vi "Reaction.vi"(8 "Size (m)":cluster{"Width":sgl, "Height":sgl}={"Width"=nan, "Height"=nan} caption="Size (m) (NaN=no change)" {"Height" format="%.2p"; "Width" format="%.2p"}, 9 "Center coordinates (m)":cluster{"Xc":sgl, "Yc":sgl}={"Xc"=nan, "Yc"=nan} caption="Center coordinates (m) (NaN=no change)" {"Yc" format="%.2p"; "Xc" format="%.2p"}, 10 "XYData":sgl[][](array[numeric]) format="%#_5p", 11 "Application ref in":refnum<vi>) -> (0 "rollout":dbl[](array[numeric]), 1 "Boolean":bool, 2 "Data":sgl[][](array[numeric]) format="%#_5p", 3 "Application ref out":refnum<vi>)   [LabVIEW 2020]
uses:
  <userlib>/Nanonis Prog Interface V5/Nanonis Prog Interface.lvlib
panel:
  in  "array 2":dbl[](array[numeric])=[1.0, 2.0]
  in  "Python version":string="3.6"
  in  "module path":path=path "D:/Git repo/pythonProject/STM_Python_Modules/RxnClass.py"
  in  "Python version 4":string="3.6"
  in  "module path 4":path=path "D:/Git repo/pythonProject/STM_Python_Modules/KpDet.py"
  in  "array":dbl[](array[numeric])=[1.0, 2.0]
  out "Error out":errorcluster
  in  "error in (no error)":errorcluster
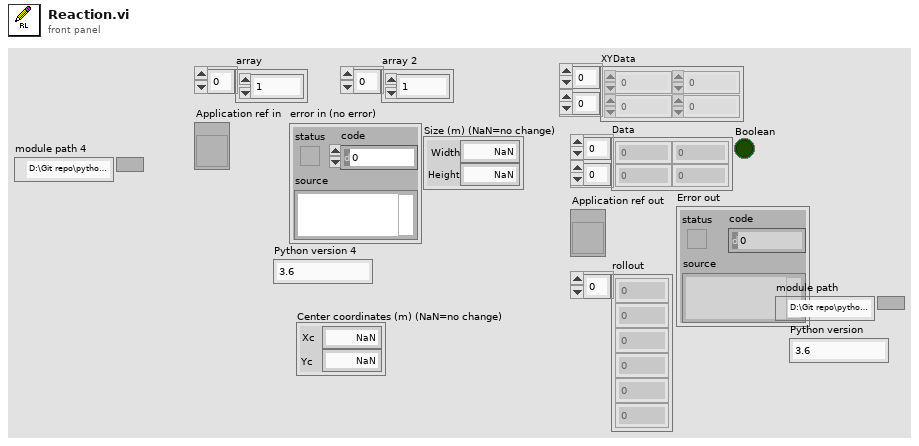
[diagram p1: front panel]
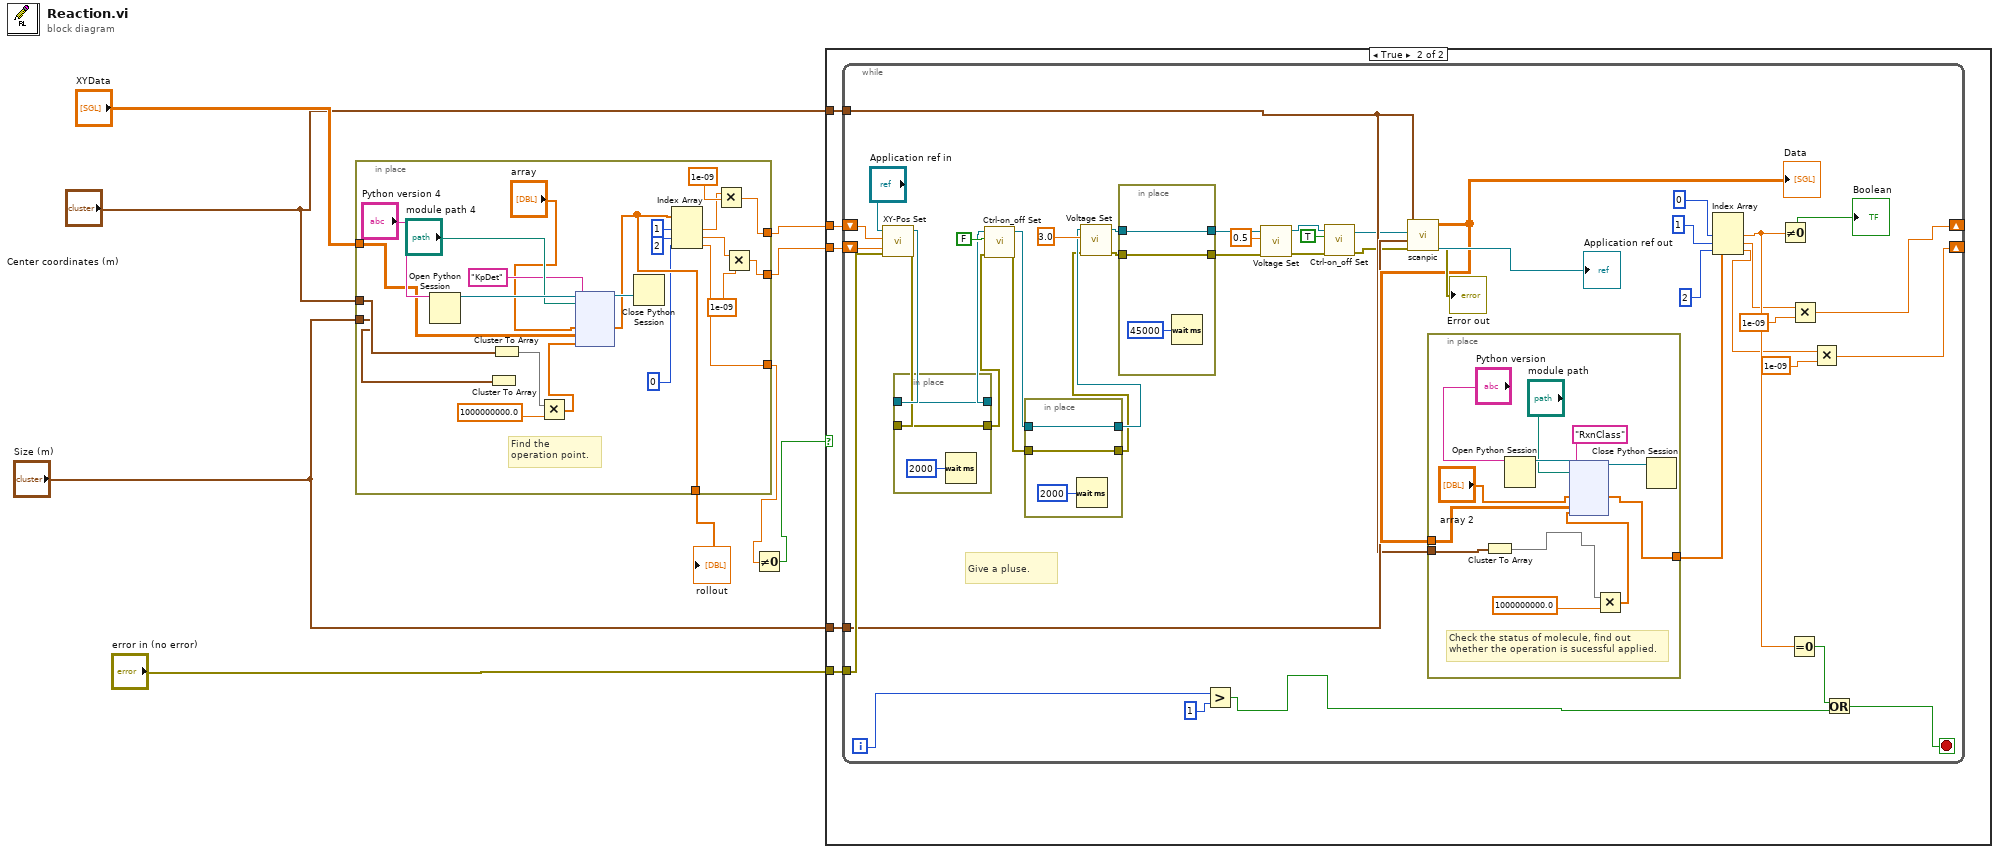
[diagram p0: block diagram]
diagram:
  n1 = in-place {
    in-place-border: "XYData" -> [w24]
    in-place-border: "Size (m)" -> [w21]
    in-place-border: [w13] -> w4
    in-place-border: [w10] -> w3
    in-place-border: [w23] -> w6
    in-place-border: "Center coordinates (m)" -> [w22]
    in-place-border: [w19] -> w2
    # "Find the operation point."
    n2 = Open Python Session(python version="Python version 4") -> (session out=w30:refnum<k35>)  [unwired: 2 in, 1 out]
    n3 = Cluster To Array(cluster=w21) -> ()  [unwired: 1 out]
    n4 = Cluster To Array(cluster=w22) -> (array=w17:sgl[])
    n5 = Multiply(x=w17, y=1000000000.0) -> (x*y=w16:dbl[])
    n6 = node(w30, "module path 4", "KpDet" ("function name"), "array", w24, w16) -> (w29:refnum<k35>, w23:dbl[])  [unwired: 3 in, 3 out]
    n7 = Close Python Session(session in=w29) -> ()  [unwired: 1 in, 1 out]
    n8 = Index Array(array=w23, index #1=1 ("index"), index #2=2 ("index"), index #3=0 ("index")) -> (element #1=w14:dbl, element #2=w11:dbl, element #3=w19:dbl)
    n9 = Multiply(x=w14, y=1e-09) -> (x*y=w13:dbl)
    n10 = Multiply(x=w11, y=1e-09) -> (x*y=w10:dbl)
  }
  "rollout" <- w6
  n11 = Not Equal To 0?(x=w2) -> (x != 0?=w1:bool)
  n12 = case shown="True" w1 {
    tunnel: "error in (no error)" -> [_ w37]
    tunnel: "Size (m)" -> [_ w36]
    tunnel: "Center coordinates (m)" -> [_ w35]
    tunnel: w4 -> [_ w34]
    tunnel: w3 -> [_ w33]
    frame False {
    }
    frame True {
      n13 = while {
        tunnel: w37 -> [w82]
        tunnel: w36 -> [w72]
        tunnel: w35 -> [w71]
        shift-right: [w46] -> _
        shift-left: w34 -> [w59]
        shift-right: [w48] -> _
        shift-left: w33 -> [w58]
        i -> [w55]
        stop <- w53 stop-if-true
        # "Give a pluse."
        n14 = call <userlib>:"XY-Pos Set.vi"("error in (no error)"=w82, "Y (m)"=w58, "X (m)"=w59, "Application ref in"="Application ref in") -> ("error out"=w43:errorcluster, "Application ref out"=w45:refnum<vi>)  [unwired: 4 in]
        n15 = in-place {
          in-place-border: w45 -> [w88]
          in-place-border: w43 -> [w89]
          in-place-border: [w89] -> w42
          in-place-border: [w88] -> w44
          n16 = Wait (ms)(milliseconds to wait=u32 2000) -> ()  [unwired: 1 out]
        }
        n17 = call <userlib>:"Ctrl-on_off Set.vi"("error in (no error)"=w42, "Z Controller ON/OFF"=FALSE, "Application ref in"=w44) -> ("error out"=w39:errorcluster, "Application ref out"=w41:refnum<vi>)  [unwired: 7 in]
        n18 = in-place {
          in-place-border: w41 -> [w85]
          in-place-border: w39 -> [w86]
          in-place-border: [w86] -> w38
          in-place-border: [w85] -> w40
          n19 = Wait (ms)(milliseconds to wait=u32 2000) -> ()  [unwired: 1 out]
        }
        n20 = call <userlib>:"Voltage Set.vi"("Error in (no error)"=w38, "Bias (V)"=sgl 3.0, "Application ref in"=w40) -> ("Error out"=w79:errorcluster, "Application ref out"=w80:refnum<vi>)  [unwired: 7 in]
        n21 = in-place {
          in-place-border: w80 -> [w103]
          in-place-border: w79 -> [w104]
          in-place-border: [w104] -> w77
          in-place-border: [w103] -> w78
          n22 = Wait (ms)(milliseconds to wait=u32 45000) -> ()  [unwired: 1 out]
        }
        n23 = Greater?(x=w55, y=1) -> (0:w47:bool)
        n24 = call <userlib>:"Voltage Set.vi"("Error in (no error)"=w77, "Bias (V)"=sgl 0.5, "Application ref in"=w78) -> ("Error out"=w67:errorcluster, "Application ref out"=w68:refnum<vi>)  [unwired: 7 in]
        n25 = call <userlib>:"Ctrl-on_off Set.vi"("error in (no error)"=w67, "Z Controller ON/OFF"=TRUE, "Application ref in"=w68) -> ("error out"=w65:errorcluster, "Application ref out"=w66:refnum<vi>)  [unwired: 7 in]
        n26 = call "scanpic.vi"("error in (no error)"=w65, "Size (m)"=w72, "Application ref in"=w66, "Center coordinates (m)"=w71) -> ("Error out"=→"Error out":errorcluster, "Application ref out"=→"Application ref out":refnum<vi>, "Data"=w73:sgl[][])  [unwired: 5 in]
        "Data" <- w73
        n27 = in-place {
          in-place-border: w73 -> [w96]
          in-place-border: [w95] -> w64
          in-place-border: w71 -> [w94]
          # "Check the status of molecule, find out whether the operation is sucessful applied."
          n28 = Cluster To Array(cluster=w94) -> (array=w91:sgl[])
          n29 = Open Python Session(python version="Python version") -> (session out=w101:refnum<k35>)  [unwired: 2 in, 1 out]
          n30 = Multiply(x=w91, y=1000000000.0) -> (x*y=w90:dbl[])
          n31 = node(w101, "module path", "RxnClass" ("function name"), "array 2", w96, w90) -> (w100:refnum<k35>, w95:dbl[])  [unwired: 3 in, 3 out]
          n32 = Close Python Session(session in=w100) -> ()  [unwired: 1 in, 1 out]
        }
        n33 = Index Array(array=w64, index #1=0, index #2=1, index #3=2) -> (element #1=w57:dbl, element #2=w50:dbl, element #3=w49:dbl)
        n34 = Not Equal To 0?(x=w57) -> (x != 0?=→"Boolean":bool)
        n35 = Equal To 0?(x=w57) -> (x = 0?=w56:bool)
        n36 = Multiply(x=w50, y=1e-09) -> (x*y=w46:dbl)
        n37 = Multiply(x=w49, y=1e-09) -> (x*y=w48:dbl)
        n38 = Or(x=w56, y=w47) -> (x .or. y?=w53:bool)
      }
    }
  }
